vi "Invite.vi"(0 "DataIn":T1={"Quem Joga"="", "Tabuleiro"={"(0,0)"="", "(1,0)"="", "(0,1)"="", "(1,1)"="", "(2,0)"="", "(1,2)"="", "(2,2)"="", "(0,2)"="", "(2,1) "=""}, "GameOption"=enum."Multiplayer local", "Turno"=FALSE, "Player"="", "Player 1"="", "Player 2"="", "Dificuldade"=enum."Easy", "Table"=[], "Row"=0, "Aceitar Convite"=FALSE, "Inviter line"=0, "diretório"=path "", "Logout - panel close"=FALSE, "StartGame"=FALSE, "MatchData.lvclass"=refnum, "GameMode"=enum."Single Easy"}) -> (7 "DataOut":T1={"Quem Joga"="", "Tabuleiro"={"(0,0)"="", "(1,0)"="", "(0,1)"="", "(1,1)"="", "(2,0)"="", "(1,2)"="", "(2,2)"="", "(0,2)"="", "(2,1) "=""}, "GameOption"=enum."Multiplayer local", "Turno"=FALSE, "Player"="", "Player 1"="", "Player 2"="", "Dificuldade"=enum."Easy", "Table"=[], "Row"=0, "Aceitar Convite"=FALSE, "Inviter line"=0, "diretório"=path "", "Logout - panel close"=FALSE, "StartGame"=FALSE, "MatchData.lvclass"=refnum, "GameMode"=enum."Single Easy"})   [LabVIEW 2018]
uses:
  controls/DataIn.ctl
  MatchDataClasses/MatchData/MatchData.lvclass
  controls/Tabuleiro.ctl
  controls/GameOption.ctl
  controls/Table.ctl
  <userlib>/_SmartBalloon/Balloon Generic/Aesthetics.ctl
  <userlib>/_SmartBalloon/API/SmartBalloon Library.lvclass/SmartBalloon Library.ctl
  <userlib>/_SmartBalloon/Balloon Generic/Balloon.lvclass/Balloon.ctl
  <userlib>/_SmartBalloon/Balloon Generic/Read Text.vi
  <userlib>/_SmartBalloon/API/Read Events.vi
  <userlib>/_SmartBalloon/Balloon/Text Balloon.lvclass
  C:/Program Files (x86)/National Instruments/LabVIEW 2018/user.lib/_SmartBalloon/Balloon Generic/Balloon.lvclass
  <vilib>/Utility/file.llb/Read Delimited Spreadsheet (string).vi
  <userlib>/_SmartBalloon/Balloon Generic/Balloon.lvclass
  <userlib>/_SmartBalloon/API/SmartBalloon Library.lvclass
panel:
  out "Click Time Stamp":timestamp
  out "Clicked Balloon Title":string
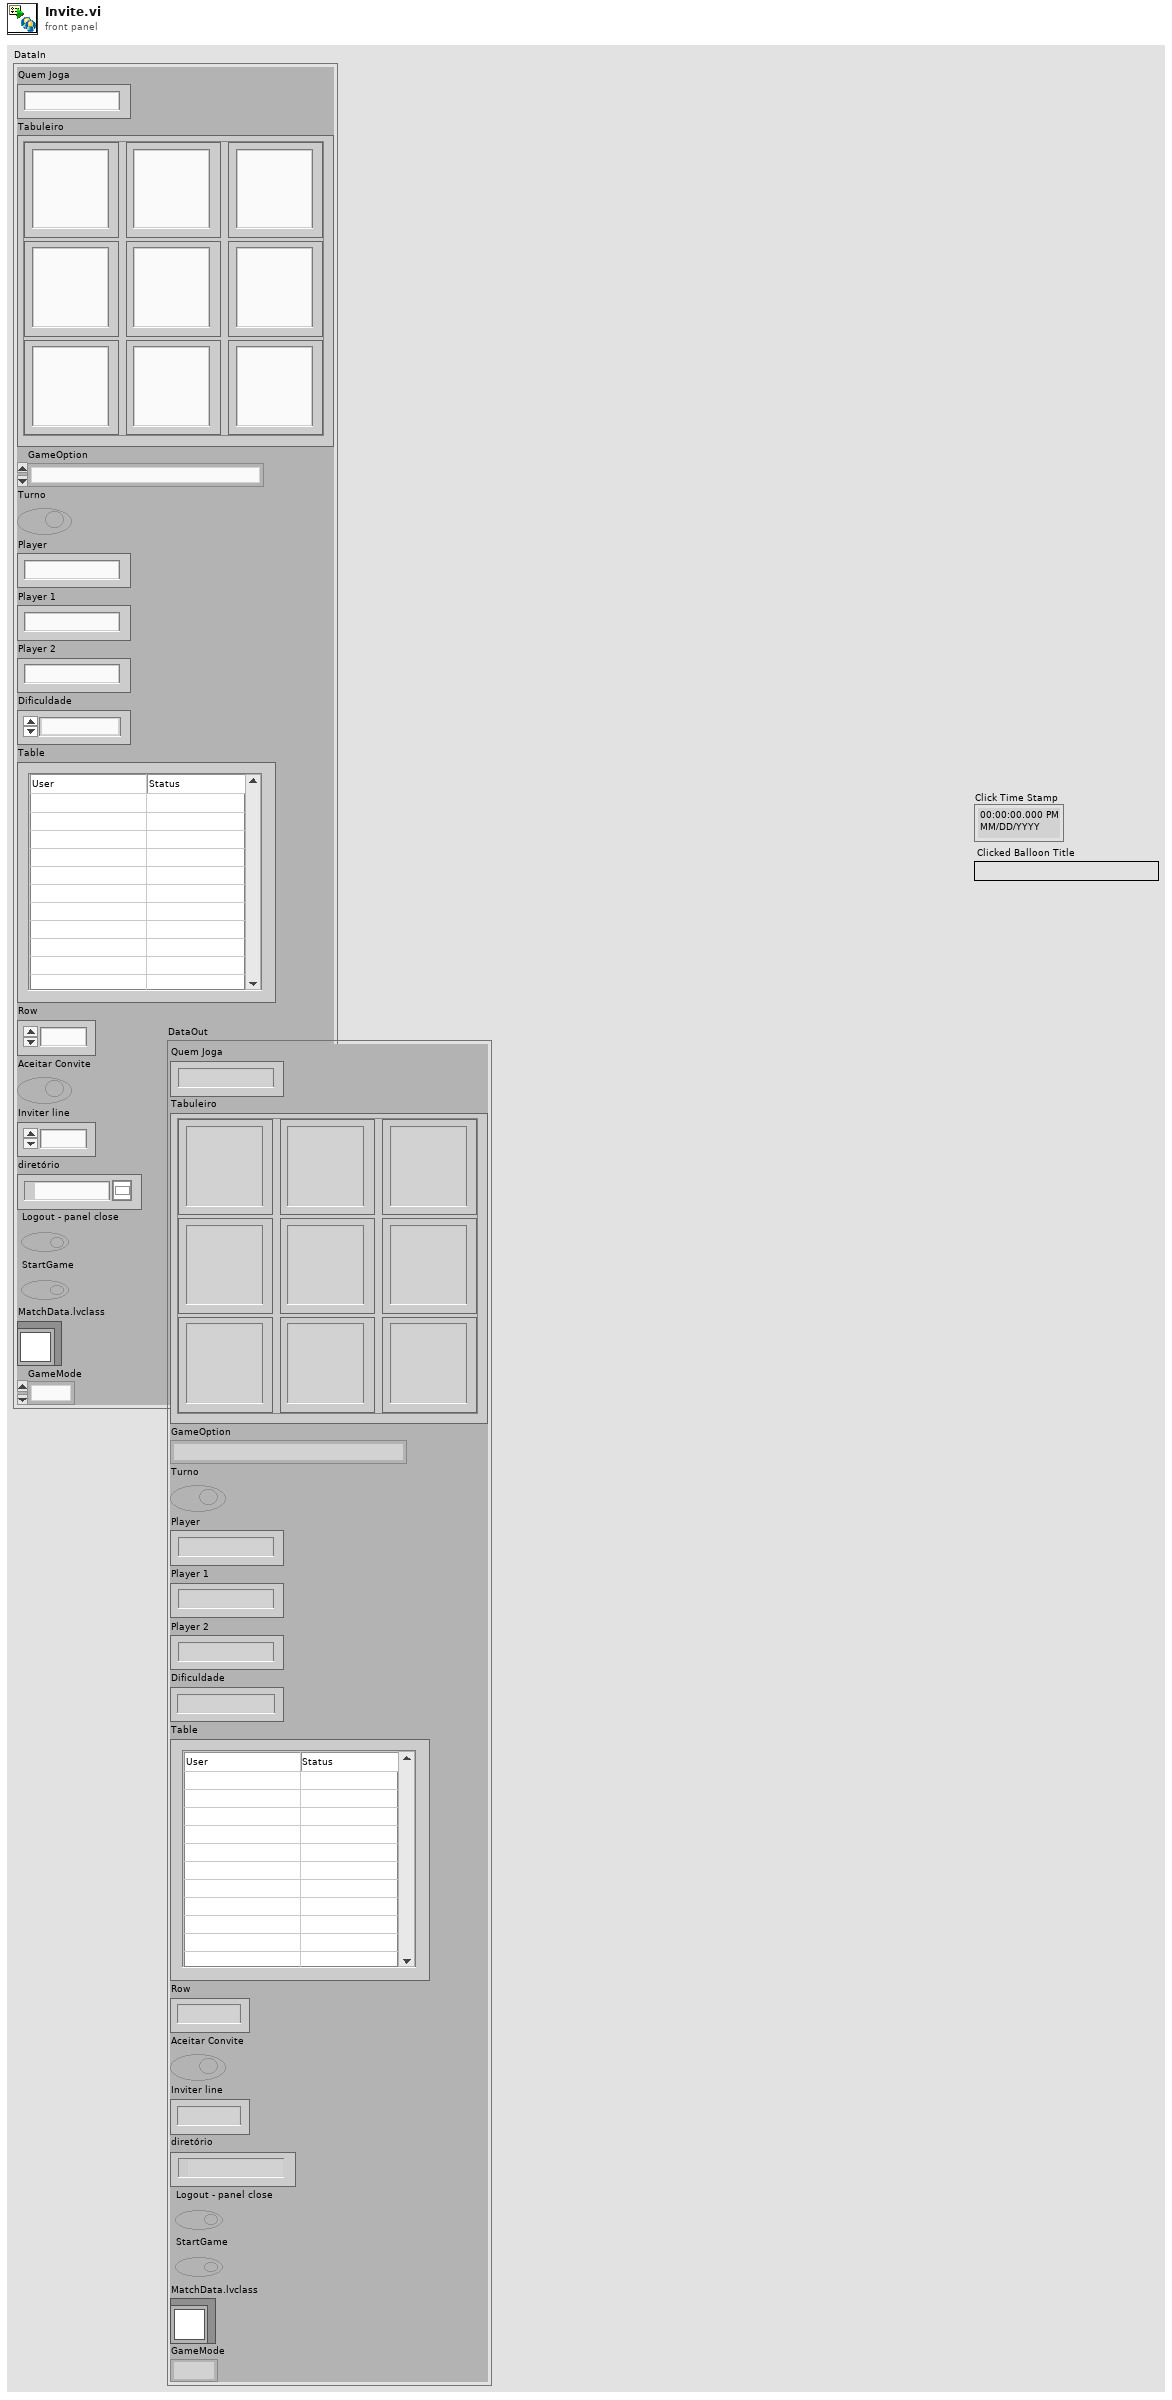
[diagram p1: front panel]
types:
  T1 = typedef "DataIn.ctl" = cluster{"Quem Joga":string, "Tabuleiro":T2, "GameOption":T3, "Turno":bool, "Player":string, "Player 1":string, "Player 2":string, "Dificuldade":enum16{"Easy", "Medium", "Hard"}, "Table":T4, "Row":u32, "Aceitar Convite":bool, "Inviter line":u32, "diretório":path, "Logout - panel close":bool, "StartGame":bool, "MatchData.lvclass":refnum<class "MatchData.lvclass">, "GameMode":enum16{"Single Easy", "Single Medium", "Single Hard", "Local", "Remote"}}
  T2 = typedef "Tabuleiro.ctl" = cluster{"(0,0)":string, "(1,0)":string, "(0,1)":string, "(1,1)":string, "(2,0)":string, "(1,2)":string, "(2,2)":string, "(0,2)":string, "(2,1) ":string}
  T3 = typedef "GameOption.ctl" = enum16{"Single Player", "Multiplayer local", "Multiplayer remoto", "Wait for Event", "Initialize", "Stop"}
  T4 = typedef "Table.ctl" = string[][]
  T5 = typedef "Balloon Engine.lvlib/Balloon.lvclass/Aesthetics.ctl" = cluster{"Colors":cluster{"Font Color":u32, "Panel Color":u32}, "Display Time (ms)":i32}
  T6 = typedef "Balloon Engine.lvlib/Balloon Display Controller.lvclass/Controller Events.ctl" = cluster{"BalloonError Event":refnum<user-event>, "BalloonClicked Event":refnum<user-event>}
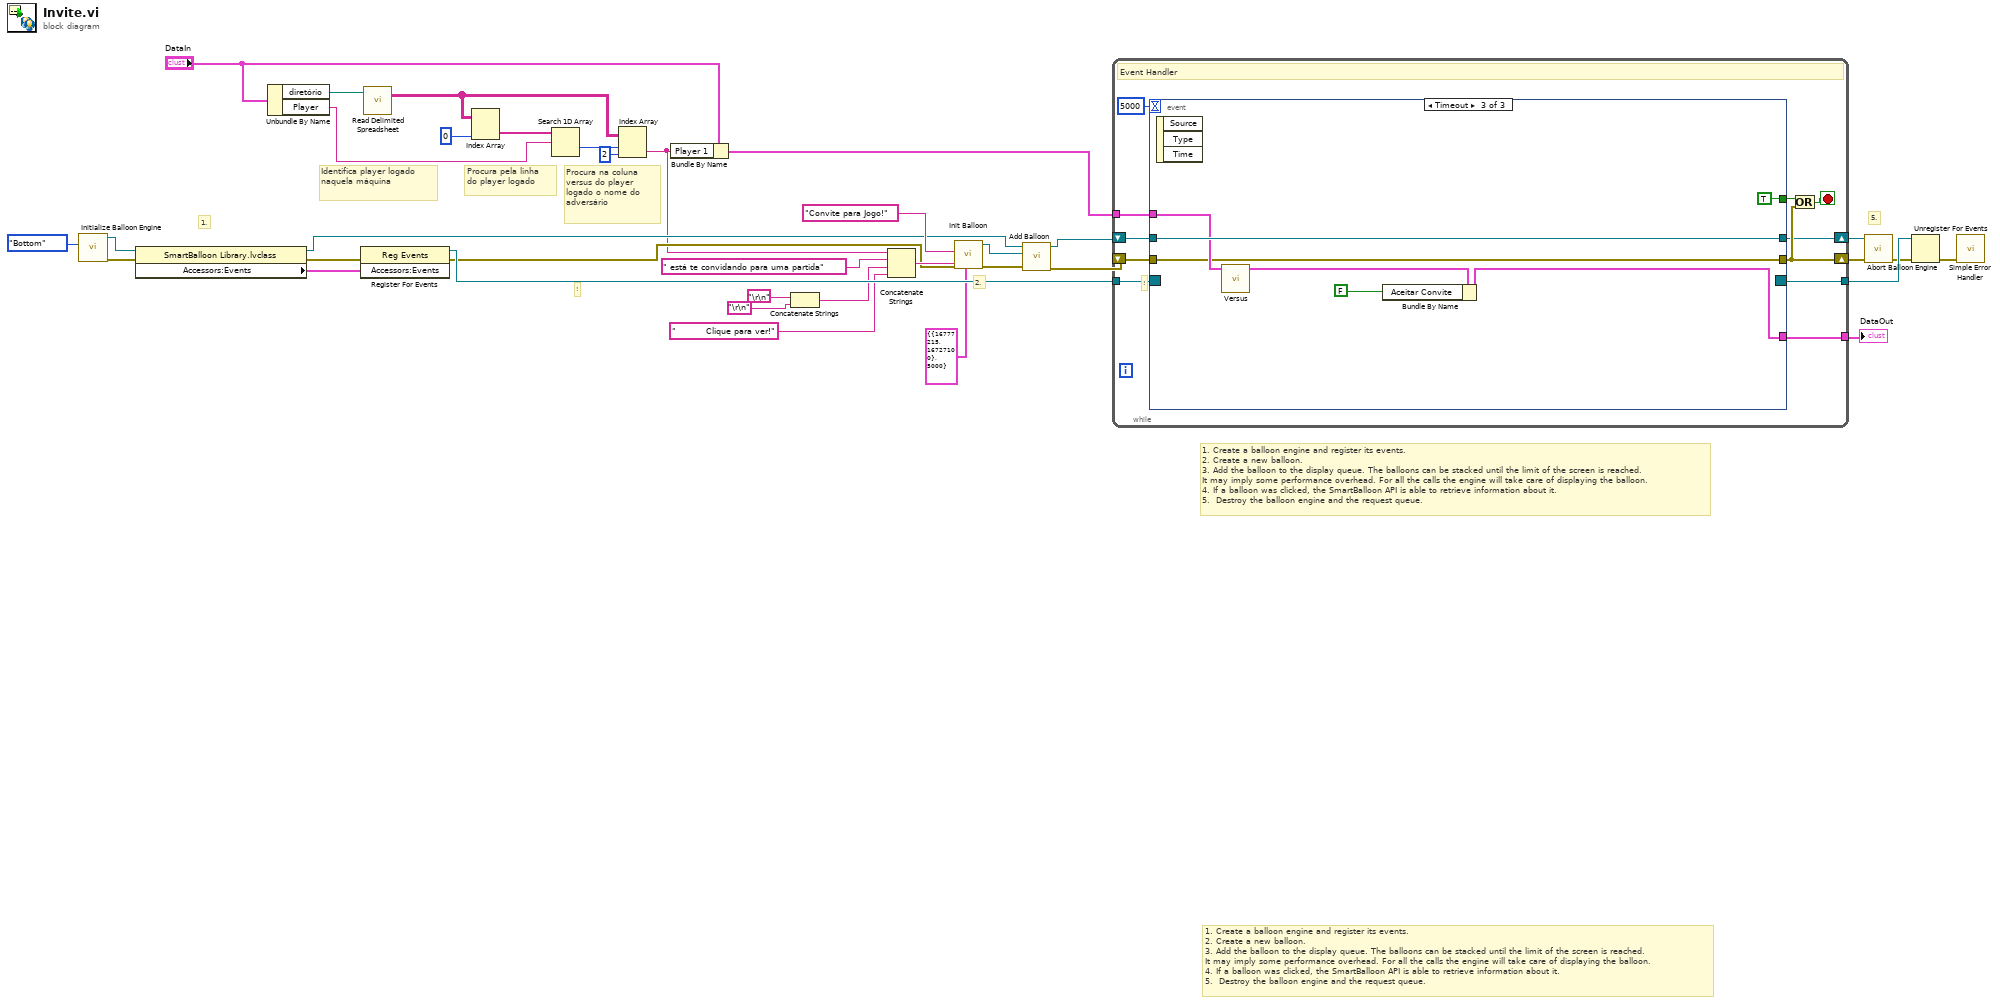
[diagram p0: block diagram]
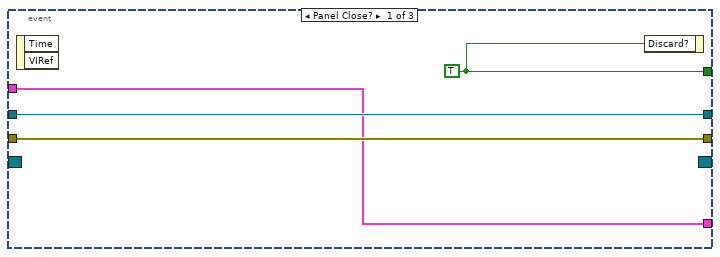
[diagram p2: hidden frame]
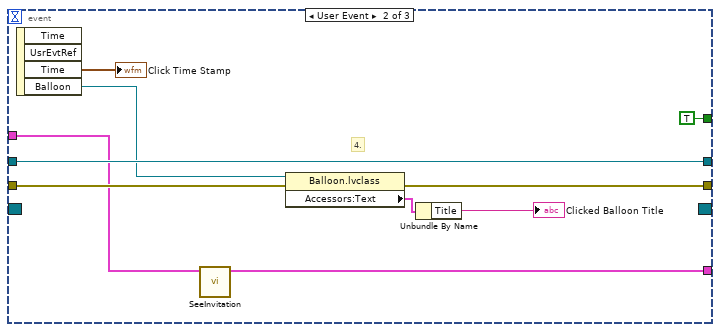
[diagram p3: hidden frame]
diagram:
  # "Procura na coluna versus do player logado o nome do adversário"
  # "Procura pela linha do player logado"
  # "Identifica player logado naquela máquina"
  # "2."
  # "!"
  # "1. Create a balloon engine and register its events.\n2. Create a new balloon.\n3. Add the balloon to the display queue. The balloons can be stacked until the limit of the screen is reached. \nIt may imply some performance overhead. For all the calls the engine will take care of displaying the balloon.\n4. If a balloon was clicked, the SmartBalloon API is able to retrieve information about it.\n5.  Destroy the balloon engine and the request queue."
  # "5."
  # "1."
  # "1. Create a balloon engine and register its events.\n2. Create a new balloon.\n3. Add the balloon to the display queue. The balloons can be stacked until the limit of the screen is reached. \nIt may imply some performance overhead. For all the calls the engine will take care of displaying the balloon.\n4. If a balloon was clicked, the SmartBalloon API is able to retrieve information about it.\n5.  Destroy the balloon engine and the request queue."
  n1 = call <userlib>:"Initialize Balloon Engine.vi"("Balloon Direction"=enum16{"Top", "Bottom"}."Bottom" ("Balloon Position")) -> ("error out"=w35:errorcluster, "SmartBalloon Library.lvclass"=w33:refnum<class "SmartBalloon Library.lvclass">)  [unwired: 9 in]
  n2 = property class="SmartBalloon Library.lvclass"(reference=w33, error in=w35) -> (reference out=w13:refnum<class "SmartBalloon Library.lvclass">, error out=w36:errorcluster, "Accessors:Events"=w34:T6)
  n3 = Unbundle By Name("DataIn") -> ("diretório"=w10:path, "Player"=w7:string)
  n4 = register-events(error in=w36, w34) -> (reference out=w27:refnum<event-registration>, error out=w14:errorcluster)  [unwired: 1 in]
  n5 = call-poly <vilib>:"Read Delimited Spreadsheet.vi"("file path (dialog if empty)"=w10) -> ("all rows"=w6:string[][])  [unwired: 9 in, 5 out]
  n6 = Index Array(array=w6, index (col)=0 ("disabled index (col)")) -> (element=w8:string[])  [unwired: 1 in]
  n7 = Search 1D Array(1D array=w8, element=w7) -> (index of element=w4:i32)  [unwired: 1 in]
  n8 = Index Array(array=w6, index (row)=w4, index (col)=2 ("disabled index (col)")) -> (element=w1:string)
  n9 = Bundle By Name(cluster="DataIn", "Player 1"=w1) -> (w2:T1)
  n10 = Concatenate Strings("\r\n", "\r\n") -> (w17:string)
  n11 = Concatenate Strings(w1, " está te convidando para uma partida" ("Body"), w17, "          Clique para ver!" ("string")) -> (w22:string)
  n12 = call <userlib>:"Init Balloon.vi"("Aesthetics"=T5 {"Colors"={"Font Color"=16777215, "Panel Color"=16727100}, "Display Time (ms)"=5000} ("Balloon Settings"), "error in (no error)"=w14, "Body"=w22, "Title"="Convite para Jogo!") -> ("error out"=w24:errorcluster, "Balloon out"=w20:refnum<class "Text Balloon.lvclass">)  [unwired: 6 in]
  n13 = call <userlib>:"Add Balloon.vi"("error in (no error)"=w24, "Next Balloon"=w20, "SmartBalloon Engine Reference"=w13) -> ("error out"=w15:errorcluster, "SmartBalloon Engine Reference out"=w12:refnum<class "SmartBalloon Library.lvclass">)  [unwired: 7 in]
  n14 = while {
    shift-right: [w43] -> w28
    shift-left: w15 -> [w46]
    tunnel: w27 -> [w42]
    shift-right: [w41] -> w29
    shift-left: w12 -> [w45]
    tunnel: [w40] -> w32
    tunnel: w2 -> [w39]
    tunnel: [w38] -> w11
    stop <- w44 stop-if-true
    # "!"
    # "Event Handler"
    n15 = event shown="[2] Timeout" {
      selector: w42 -> [_ _ _]
      dyn-events: [_ _ _] -> w40
      timeout: 5000 -> [_ _ _]
      tunnel: [w51 TRUE ("Discard?") TRUE ("Discard?")] -> w47
      tunnel: [w50 w59 w62] -> w43
      tunnel: w46 -> [w50 w55 w62]
      tunnel: w45 -> [w49 w58 w67]
      tunnel: [w49 w58 w67] -> w41
      tunnel: w39 -> [w48 w54 w64]
      tunnel: [w48 w53 w66] -> w38
      event Panel Close? {
        w51 = TRUE ("Discard?")
        n16 = event-data() -> ()  [unwired: 1 in, 2 out]
        n17 = event-data("Discard?"=w51) -> ()  [unwired: 1 in, 1 out]
      }
      event User Event {
        # "4."
        n18 = event-data() -> ("Time"=→"Click Time Stamp":timestamp, "Balloon"=w56:refnum<class "Balloon.lvclass">)  [unwired: 1 in, 2 out]
        n19 = call "SeeInvitation.vi"("DataIn"=w54) -> ("DataOut"=w53:T1)  [unwired: 10 in]
        n20 = property class="Balloon.lvclass"(reference=w56, error in=w55) -> (error out=w59:errorcluster, "Accessors:Text"=w61:cluster{"Title":string, "Body":string})  [unwired: 1 out]
        n21 = Unbundle By Name(w61) -> ("Title"=→"Clicked Balloon Title":string)
      }
      event Timeout {
        n22 = event-data() -> ()  [unwired: 1 in, 3 out]
        n23 = call "Versus.vi"("DataIn"=w64) -> ("DataOut"=w63:T1)  [unwired: 10 in]
        n24 = Bundle By Name(cluster=w63, "Aceitar Convite"=FALSE) -> (w66:T1)
      }
    }
    n25 = Or(x=w47, y=w43) -> (x .or. y?=w44:bool)
  }
  "DataOut" <- w11
  n26 = call <userlib>:"Abort Balloon Engine.vi"("error in (no error)"=w28, "SmartBalloon Engine Reference"=w29) -> ("error out"=w30:errorcluster)  [unwired: 9 in]
  n27 = Unregister For Events(event registration refnum=w32, error in=w30) -> (error out=w31:errorcluster)
  n28 = call <vilib>:"Simple Error Handler.vi"("error in (no error)"=w31) -> ()  [unwired: 4 in, 5 out]
